vi "Initialize Manager.vi"(8 "error in (no error)":errorcluster, 11 "CIF_Manager_UI in":refnum<class "CIF_Manager_UI.lvclass">) -> (0 "error out":errorcluster, 3 "CIF_Manager_UI out":refnum<class "CIF_Manager_UI.lvclass">)   [LabVIEW 2021, in "CIF_Manager_UI.lvclass"]
uses:
  CIF_Manager_UI.lvclass
  CIF_Manager_UI.lvclass/CIF_Manager_UI.ctl
  <vilib>/gRPC/LabVIEW gRPC Library/Shared/grpcId.ctl
  <vilib>/gRPC/LabVIEW gRPC Library/grpc-lvsupport-release.lvlib
  CIFPluginManager/typedef/New Connection Event Data.ctl
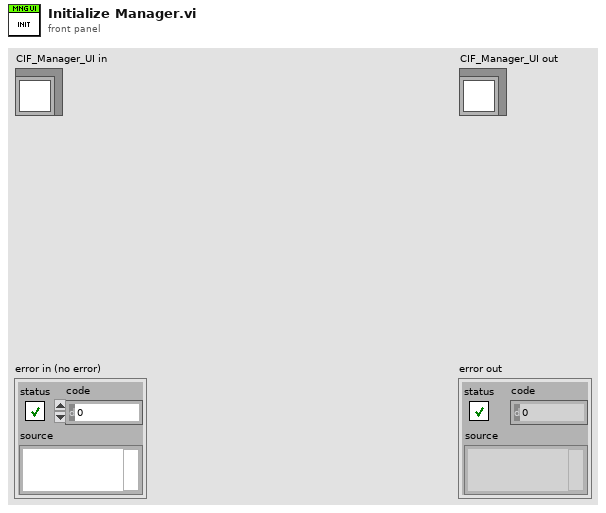
[diagram p1: front panel]
types:
  T1 = typedef "CIF_Manager_UI.lvclass/New Connection Event Data.ctl" = cluster{"Manager gRPC ID":T2, "IP Address":string, "Connected":bool}
  T2 = typedef "grpc-lvsupport-release.lvlib/grpcId.ctl" = u64
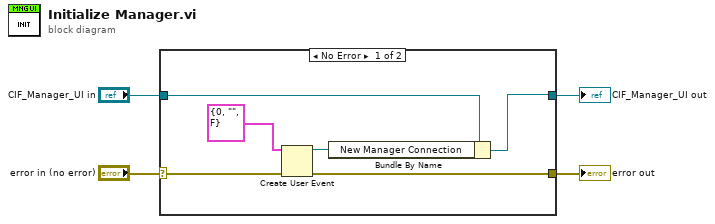
[diagram p0: block diagram]
diagram:
  n1 = case shown="No Error" "error in (no error)" {
    selector: "error in (no error)" -> [w6 w12]
    tunnel: [w5 w12] -> w3
    tunnel: [w7 w11] -> w1
    tunnel: "CIF_Manager_UI in" -> [w9 w11]
    frame No Error {
      n2 = Create User Event(user event datatype=T1 {"Manager gRPC ID"=0, "IP Address"="", "Connected"=FALSE} ("New Connection"), error in=w6) -> (user event=w8:refnum<user-event>, error out=w5:errorcluster)
      n3 = Bundle By Name(cluster=w9, "New Manager Connection"=w8) -> (w7:refnum<class "CIF_Manager_UI.lvclass">)
    }
    frame Error {
    }
  }
  "error out" <- w3
  "CIF_Manager_UI out" <- w1
